vi "Read Endpoint invoked .vi"(8 "error in (no error)":errorcluster, 11 "JsonEvents in":refnum<class "JsonEvents.lvclass">) -> (0 "error out":errorcluster, 2 "Endpoint invoked":refnum<user-event>, 3 "JsonEvents out":refnum<class "JsonEvents.lvclass">)   [LabVIEW 2020, in "wamplv.lvlib" / "JsonEvents.lvclass"]
uses:
  JsonEvents.lvclass
  WAMP Client/API/TypeDefs/INVOCATION payload.ctl
  Invocation Request ID/Invocation Request ID.lvclass
  JsonEvents.lvclass/JsonEvents.ctl
  WAMP Client/WAMP Client.lvclass
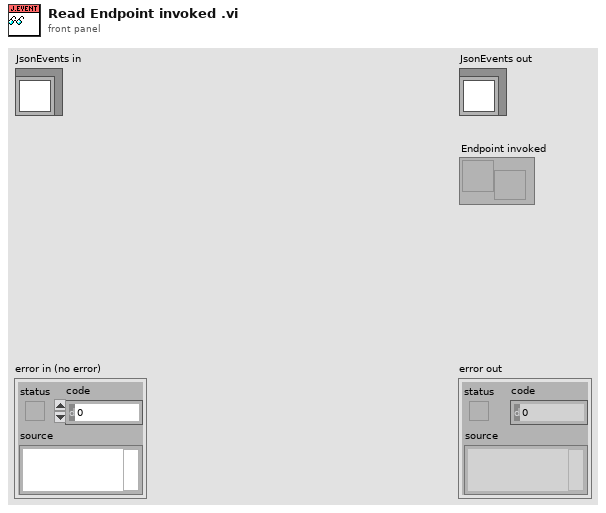
[diagram p1: front panel]
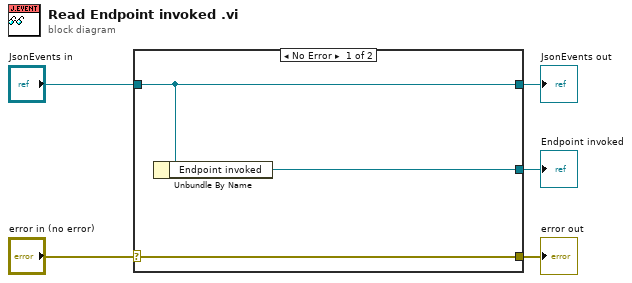
[diagram p0: block diagram]
diagram:
  n1 = case shown="No Error" "error in (no error)" {
    selector: "error in (no error)" -> [w8 w9]
    tunnel: [w8 w9] -> w4
    tunnel: [w7 w10] -> w2
    tunnel: "JsonEvents in" -> [w7 w10]
    tunnel: [w6 _] -> w1
    frame No Error {
      n2 = Unbundle By Name(w7) -> ("Endpoint invoked"=w6:refnum<user-event>)
    }
    frame Error {
    }
  }
  "error out" <- w4
  "JsonEvents out" <- w2
  "Endpoint invoked" <- w1
